vi "SimpleVisionAlign.vi"(8 "Manual Turn":dbl, 9 "Target Offset":dbl=-4.3501129150390625, 10 "Gyro Angle":dbl=-17.65, 11 "Throttle":dbl=-0.0) -> (2 "Right Power":dbl=0.10095338752954246, 3 "Left Power":dbl=-0.10095338752954246)   [LabVIEW 2019]
uses:
  <vilib>/addons/control/pid/pid.llb/PID (DBL).vi
  <vilib>/addons/control/pid/NI_PID_pid.lvlib
  Drive/Implementation/Drive Published Globals.vi
  <vilib>/Rock Robotics/Network Tables/NT Read Number.vi
panel:
  in  "Manual Turn Divisor":dbl=5.0
  in  "PID gains":T1={"proportional gain (Kc)"=0.03, "integral time (Ti, min)"=0.0, "derivative time (Td, min)"=0.0003} {"derivative time (Td, min)" format="%.5f"; "integral time (Ti, min)" format="%.3f"; "proportional gain (Kc)" format="%.3f"}
  in  "output range":cluster{"output high":dbl, "output low":dbl}={"output high"=0.5, "output low"=-0.5} {"output low" format="%.2f"; "output high" format="%.2f"}
  in  "Latency Compensator":i32=4
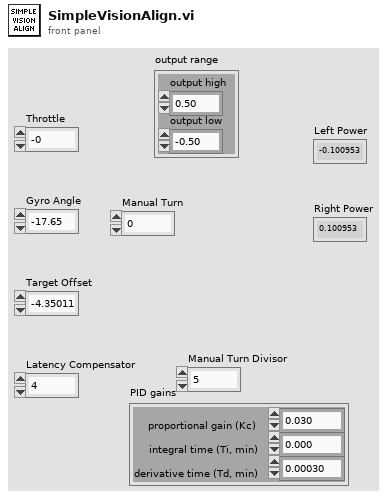
[diagram p1: front panel]
types:
  T1 = cluster{"proportional gain (Kc)":dbl, "integral time (Ti, min)":dbl, "derivative time (Td, min)":dbl}
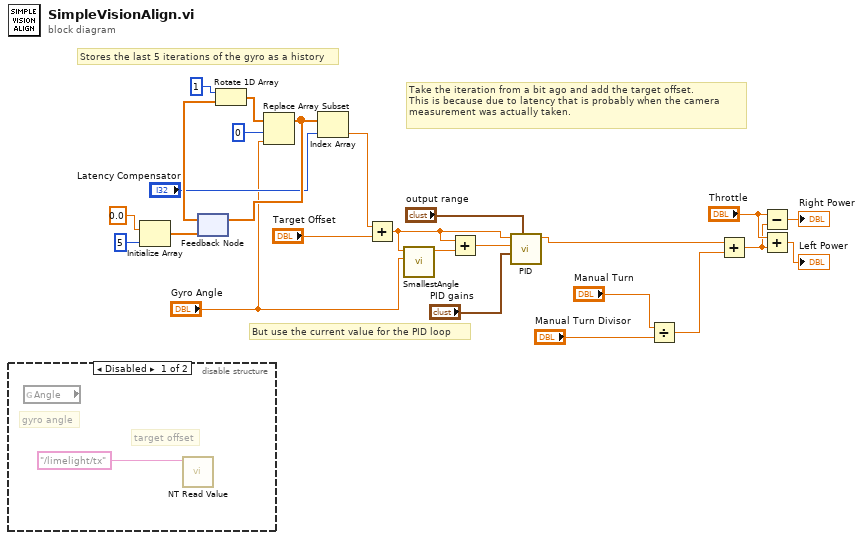
[diagram p0: block diagram]
diagram:
  # "But use the current value for the PID loop"
  # "Take the iteration from a bit ago and add the target offset.\nThis is because due to latency that is probably when the camera\nmeasurement was actually taken."
  # "Stores the last 5 iterations of the gyro as a history"
  n1 = disable-structure shown="Disabled" {
    frame Disabled {
      # "target offset"
      # "gyro angle"
      n2 = global read "Drive Published Globals.vi" "Angle"() -> ()  [unwired: 1 out]
      n3 = call-poly <vilib>:"NT Read Value.vi"("Name"="/limelight/tx") -> ()  [unwired: 9 in, 2 out]
    }
    frame Enabled {
    }
  }
  n4 = Initialize Array(0.0 ("element"), 5 ("dimension size")) -> (w16:dbl[])
  n5 = feedback #1(w16) -> (w13:dbl[])
  n6 = Rotate 1D Array(1:w13, 2:1 ("n")) -> (0:w11:dbl[])
  n7 = Replace Array Subset(array=w11, new element="Gyro Angle", index=0) -> (w9:dbl[])
  n8 = feedback-in #1(w9) -> ()
  n9 = Index Array(array=w9, index="Latency Compensator") -> (element=w7:dbl)
  n10 = Add(x=w7, y="Target Offset") -> (x+y=w18:dbl)
  n11 = call "SmallestAngle.vi"("Angle B"="Gyro Angle", "Angle A"=w18) -> ("Smallest A to B"=w19:dbl)  [unwired: 9 in]
  n12 = Add(x=w18, y=w19) -> (x+y=w17:dbl)
  n13 = call-poly <vilib>:"PID.vi"("output range"="output range", "PID gains"="PID gains", "process variable"=w17, "setpoint"=w18) -> ("output"=w4:dbl)  [unwired: 6 in, 1 out]
  n14 = Divide(x="Manual Turn", y="Manual Turn Divisor") -> (x/y=w3:dbl)
  n15 = Add(x=w4, y=w3) -> (x+y=w2:dbl)
  n16 = Subtract(x="Throttle", y=w2) -> (x-y=→"Right Power":dbl)
  n17 = Add(x="Throttle", y=w2) -> (x+y=→"Left Power":dbl)
